vi "Noise-Compute Max Level.vi"(0 "Noise Params":T4, 5 "Filter XCtl":T3(xcontrol), 9 "Level":T1, 11 "error in (no error)":errorcluster, 12 "Sampling Rate (Hz)":dbl, 13 "Npts":i32) -> (6 "Max Level":dbl, 10 "Level out":T1, 15 "error out":errorcluster)   [LabVIEW 2020]
uses:
  Noise Params.ctl
  Controls/Filter XCtl/Filter XCtl.xctl
  Controls/Level XCtl/Level Data.ctl
  Controls/Level XCtl/Level Units.ctl
  <vilib>/Analysis/5stat.llb/RMS (DBL).vi
  Noise-Globals.vi
  PXI DAQ VIs/DAQ Engine VIs/PXI Globals.vi
  Utility VIs/Math VIs/Linear to dB (scalar).vi
  <vilib>/Analysis/NI_AALPro.lvlib
  Controls/Level XCtl/Level XCtl.xctl
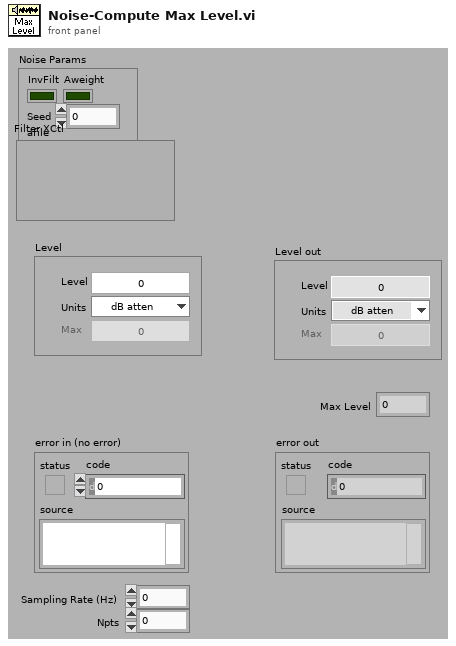
[diagram p1: front panel]
types:
  T1 = typedef "Level XCtl.xctl/Level Data.ctl" = cluster{"Level":dbl, "Units":T2, "Max":dbl, "Multiplier":dbl, "Cal File":path, "Cal":cluster{"Freq (Hz)":dbl[], "Mag (dB SPL)":dbl[], "Phase (deg)":dbl[]}}
  T2 = typedef "Level Units.ctl" = enum16{"dB atten", "dB SPL", "dB re 1 Vrms", "dB V/Hz½", "mW", "dB HL", "Volts", "dB mW"}
  T3 = cluster{"CF (kHz)":dbl, "BW (kHz)":dbl, "IIR Filter Cluster":cluster{"filter structure":enum32{"IIR 2nd Order", "IIR 4th Order"}, "Reverse Coefficients":dbl[], "Forward Coefficients":dbl[]}, "Final Filter State":dbl[], "Scale Factor":dbl, "Final Filter State 2":dbl[], "Quadrature":bool, "Type":enum16{"Lowpass", "Highpass", "Bandpass", "Bandstop", "OFF"}}
  T4 = typedef "Noise Params.ctl" = cluster{"InvFilt":bool, "Noise":dbl[], "CurPt":i32, "Aweight":bool, "Seed":i32, "afile":path}
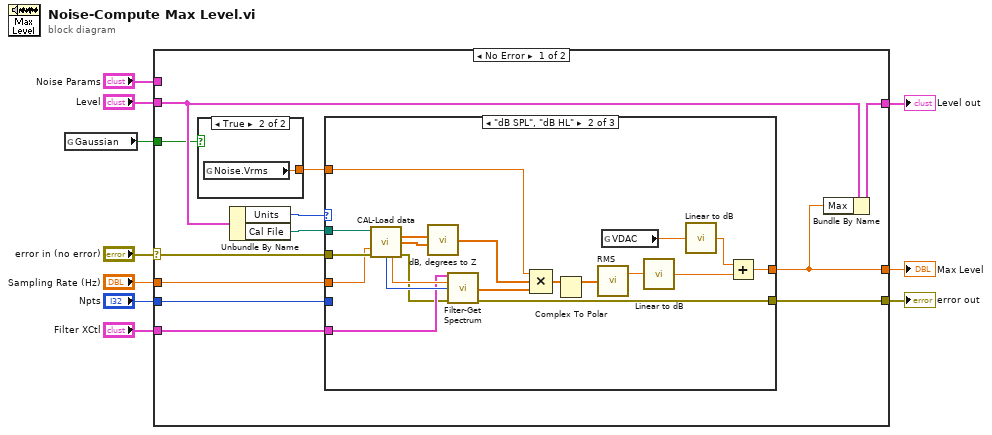
[diagram p0: block diagram]
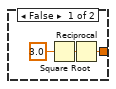
[diagram p2: hidden frame]
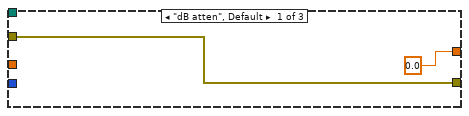
[diagram p3: hidden frame]
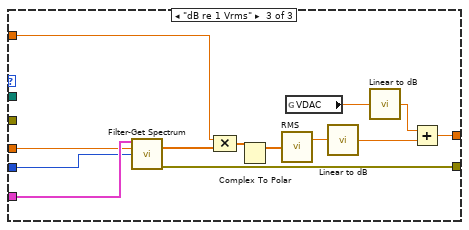
[diagram p4: hidden frame]
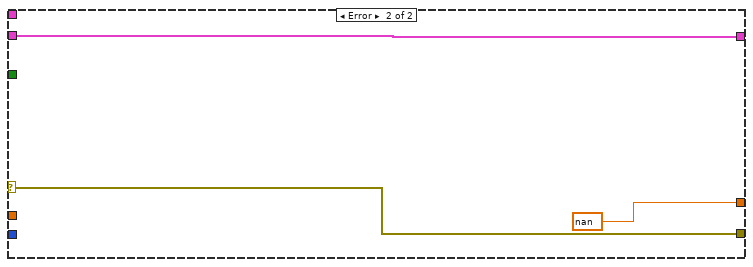
[diagram p5: hidden frame]
diagram:
  n1 = global read "Noise-Globals.vi" "Gaussian"() -> (w1:bool)
  n2 = case shown="No Error" "error in (no error)" {
    selector: "error in (no error)" -> [w22 w64]
    tunnel: "Level" -> [w17 w62]
    tunnel: "Noise Params" -> [_ _]
    tunnel: "Filter XCtl" -> [w20 _]
    tunnel: [w18 w64] -> w9
    tunnel: "Npts" -> [w21 _]
    tunnel: [w16 nan ("Reference Level")] -> w4
    tunnel: "Sampling Rate (Hz)" -> [w19 _]
    tunnel: [w15 w62] -> w2
    tunnel: w1 -> [w11 _]
    frame No Error {
      n3 = case shown="True" w11 {
        tunnel: [w25 w26] -> w12
        frame False {
          n4 = Square Root(x=3.0 ("Noise Vrms")) -> (sqrt(x)=w23:dbl)
          n5 = Reciprocal(x=w23) -> (1/x=w25:dbl)
        }
        frame True {
          n6 = global read "Noise-Globals.vi" "Noise.Vrms"() -> (w26:dbl)
        }
      }
      n7 = Unbundle By Name(w17) -> ("Units"=w14:T2, "Cal File"=w13:path)
      n8 = case shown="\"dB SPL\", \"dB HL\"" w14 {
        tunnel: w22 -> [w27 w48 _]
        tunnel: w21 -> [_ _ w50]
        tunnel: w20 -> [_ w45 w61]
        tunnel: [0.0 ("Reference Level") w42 w59] -> w16
        tunnel: w19 -> [_ w29 w51]
        tunnel: [w27 w31 w52] -> w18
        tunnel: w13 -> [_ w40 _]
        tunnel: w12 -> [_ w30 w49]
        frame "dB atten", Default {
        }
        frame "dB SPL", "dB HL" {
          n9 = call "CAL-Load data.vi"("user path"=w40, "Desired Fs (Hz)"=w29, "error in (no error)"=w48) -> ("Mag"=w39:dbl[], "Phase"=w38:dbl[], "npts"=w46:i32, "Fs (Hz)"=w47:dbl, "error out"=w44:errorcluster)  [unwired: 5 in, 3 out]
          n10 = call "dB, degrees to Z.vi"("Magnitude (dB)"=w39, "Phase (degrees)"=w38) -> ("Z"=w34:cdb[])  [unwired: 5 in]
          n11 = call "Filter-Get Spectrum.vi"("Filter"=w45, "Sampling Rate (Hz)"=w47, "Npts"=w46, "error in (no error)"=w44) -> ("spectrum"=w35:cdb[], "error out"=w31:errorcluster)  [unwired: 9 in, 1 out]
          n12 = Compound Arithmetic op=MULTIPLY(w30, w34, w35) -> (w36:cdb[])
          n13 = Complex To Polar(r * e^(i*theta)=w36) -> (r=w33:dbl[])  [unwired: 1 out]
          n14 = call-poly <vilib>:"RMS.vi"("X"=w33) -> ("rms value"=w37:dbl)  [unwired: 1 out]
          n15 = global read "PXI Globals.vi" "VDAC"() -> (w43:dbl)
          n16 = call-poly "Linear to dB.vi"("Linear"=w37) -> ("dB"=w32:dbl)
          n17 = call-poly "Linear to dB.vi"("Linear"=w43) -> ("dB"=w41:dbl)
          n18 = Add(x=w41, y=w32) -> (x+y=w42:dbl)
        }
        frame "dB re 1 Vrms" {
          n19 = call "Filter-Get Spectrum.vi"("Filter"=w61, "Sampling Rate (Hz)"=w51, "Npts"=w50) -> ("spectrum"=w55:cdb[], "error out"=w52:errorcluster)  [unwired: 10 in, 1 out]
          n20 = Compound Arithmetic op=MULTIPLY(w49, w55) -> (w56:cdb[])
          n21 = Complex To Polar(r * e^(i*theta)=w56) -> (r=w54:dbl[])  [unwired: 1 out]
          n22 = call-poly <vilib>:"RMS.vi"("X"=w54) -> ("rms value"=w57:dbl)  [unwired: 1 out]
          n23 = global read "PXI Globals.vi" "VDAC"() -> (w60:dbl)
          n24 = call-poly "Linear to dB.vi"("Linear"=w57) -> ("dB"=w53:dbl)
          n25 = call-poly "Linear to dB.vi"("Linear"=w60) -> ("dB"=w58:dbl)
          n26 = Add(x=w58, y=w53) -> (x+y=w59:dbl)
        }
      }
      n27 = Bundle By Name(cluster=w17, "Max"=w16) -> (w15:T1)
    }
    frame Error {
    }
  }
  "error out" <- w9
  "Max Level" <- w4
  "Level out" <- w2
